vi "Equals.vi"(10 "Size 输入 2":refnum<class "Size.lvclass"> caption="DNL_LabVIEW Object in", 11 "Size 输入":refnum<class "Size.lvclass"> caption="DNL_LabVIEW Object in") -> (2 "Equals":bool, 3 "Size 输出":refnum<class "Size.lvclass"> caption="DNL_LabVIEW Object out")   [LabVIEW 2011, in "Size.lvclass"]
uses:
  Size.lvclass
panel:
  out "error out":errorcluster caption="错误输出"
  in  "error in (no error)":errorcluster caption="错误输入（无错误）"
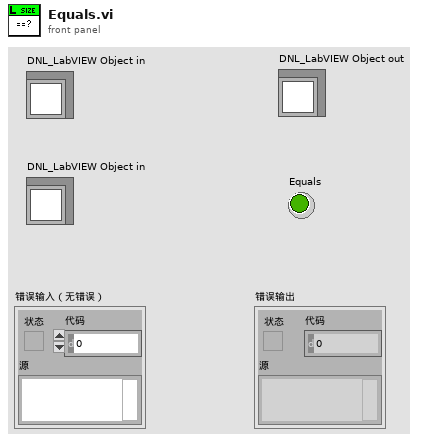
[diagram p1: front panel]
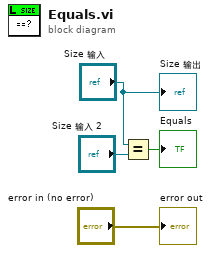
[diagram p0: block diagram]
diagram:
  n1 = Equal?(x="Size 输入", y="Size 输入 2") -> (x = y?=→"Equals":bool)
  "error out" <- "error in (no error)"
  "Size 输出" <- "Size 输入"
